vi "Actor Core.vi"(8 "error in":errorcluster, 11 "Nested in":refnum<class "FlatFieldUI.lvclass">) -> (0 "error out":errorcluster, 3 "Actor out":refnum<class "Actor.lvclass">)   [LabVIEW 2020, in "FlatFieldUI.lvlib" / "FlatFieldUI.lvclass"]
doc: "(<B>Filename</B>: Actor Framework.lvlib:Actor.lvclass:Actor Core.vi)\n\nReceives messages to the actor, reacts to them, and initiates any error handling that may shut the actor down.\n\nDescendant classes may override this VI to append parallel tasks for the actor to complete while it handles messages. Overrides use the Call Parent Method node."
uses:
  FlatFieldUI.lvclass
  <vilib>/ActorFramework/Actor/Actor.lvclass
  Displayer/Displayer/FlatField Method.ctl
  FlatFieldUI.lvclass/FlatFieldUI.ctl
  Hardware Abstraction Layer/Component/Device/Device/DataExchange.ctl
  Interface/DataListener Messages/OnDataChange Msg/OnDataChange Msg.lvclass/OnDataChange Msg.ctl
  <vilib>/ActorFramework/Message Enqueuer/Message Enqueuer.lvclass/Message Enqueuer.ctl
  <vilib>/ActorFramework/Message Enqueuer/Enqueue.vi
  Interface/DataListener Messages/OnDataChange Msg/OnDataChange Msg.lvclass
  C:/Program Files/National Instruments/LabVIEW 2020/vi.lib/ActorFramework/Message/Message.lvclass
  <vilib>/ActorFramework/Stop Msg/Stop Msg.lvclass
  <vilib>/ActorFramework/Message Priority Queue/Priority Enqueue.vi
  Hardware Abstraction Layer/Component/GenericActor/GenericActor/GenericController.lvclass
  Interface/DataListener/DataListener.lvclass
  <vilib>/vision/NI_Vision_Development_Module.lvlib
  E:/Development/DevHardSoftware/MicroscopyFramework/Model/Hardware Abstraction Layer/Component/GenericActor/GenericActor/GenericController.lvclass
  C:/Program Files/National Instruments/LabVIEW 2020/vi.lib/ActorFramework/Actor/Actor.lvclass
  E:/Development/DevHardSoftware/MicroscopyFramework/Interface/DataGenerator/DataGenerator.lvclass
  E:/Development/DevHardSoftware/MicroscopyFramework/Interface/DataListener/DataListener.lvclass
  E:/Development/DevHardSoftware/MicroscopyFramework/Interface/ErrorHandler/ErrorHandler.lvclass
  E:/Development/DevHardSoftware/MicroscopyFramework/Model/Logic Layer/FlatFieldUI/FlatFieldUI.lvclass
panel:
  in  "ZoomToFit":bool
  in  "Plot":bool
  in  "FlatFieldPath":path
  in  "DarkFieldPath":path
  in  "Save FlatField Image":bool
  in  "Save DarkField Image":bool
  in  "Method":T1 items=["Average", "Median"]
  out "XY Graph":cluster{"X":dbl, "Y":dbl}[](graph)
  in  "Show FlatField Image":bool
  in  "Show DarkField Image":bool
  out "Frames/Dark Field":dbl
  out "Frames/Flat-Field":dbl
  in  "Frames/Flat-Field":dbl
  in  "Frames/Dark Field":dbl
  in  "TakeFlatFieldImage":bool
  in  "TakeDarkFieldImage":bool
  out "RawImage":T2(plugin-control)
  in  "Flat-Field":bool
  # "* Please Take DarkField & Flat Field Images In Live Mode\n* You need to save the DarkField/FlatField images manually for post-processing"
  # "/"
  # "1."
  # "/"
  # "2."
  # "3."
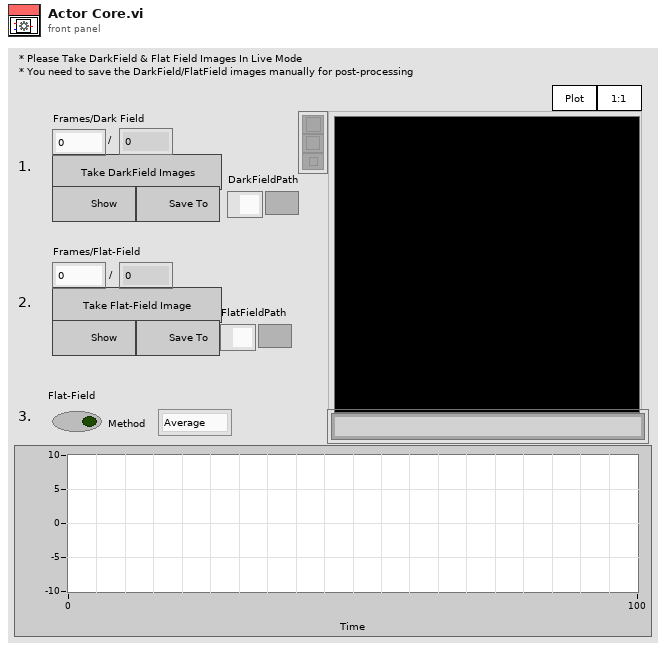
[diagram p1: front panel]
types:
  T1 = typedef "FlatFieldUI.lvlib/FlatFieldUI.lvclass/FlatField Method.ctl" = i32
  T2 = typedef "IMAQ Image.ctl" = refnum<image>
  T3 = cluster{"Stop":refnum<user-event>, "Image":refnum<user-event>}
  T4 = typedef "DataListener.lvclass/DataExchange.ctl" = cluster{"Source":string, "Destination":string, "Description":string, "value":variant}
  T5 = cluster{"Global Rectangle":i32[], "Contours":cluster{"Contour Type":u32, "ROI Type":u32, "Points":i32[]}[]}
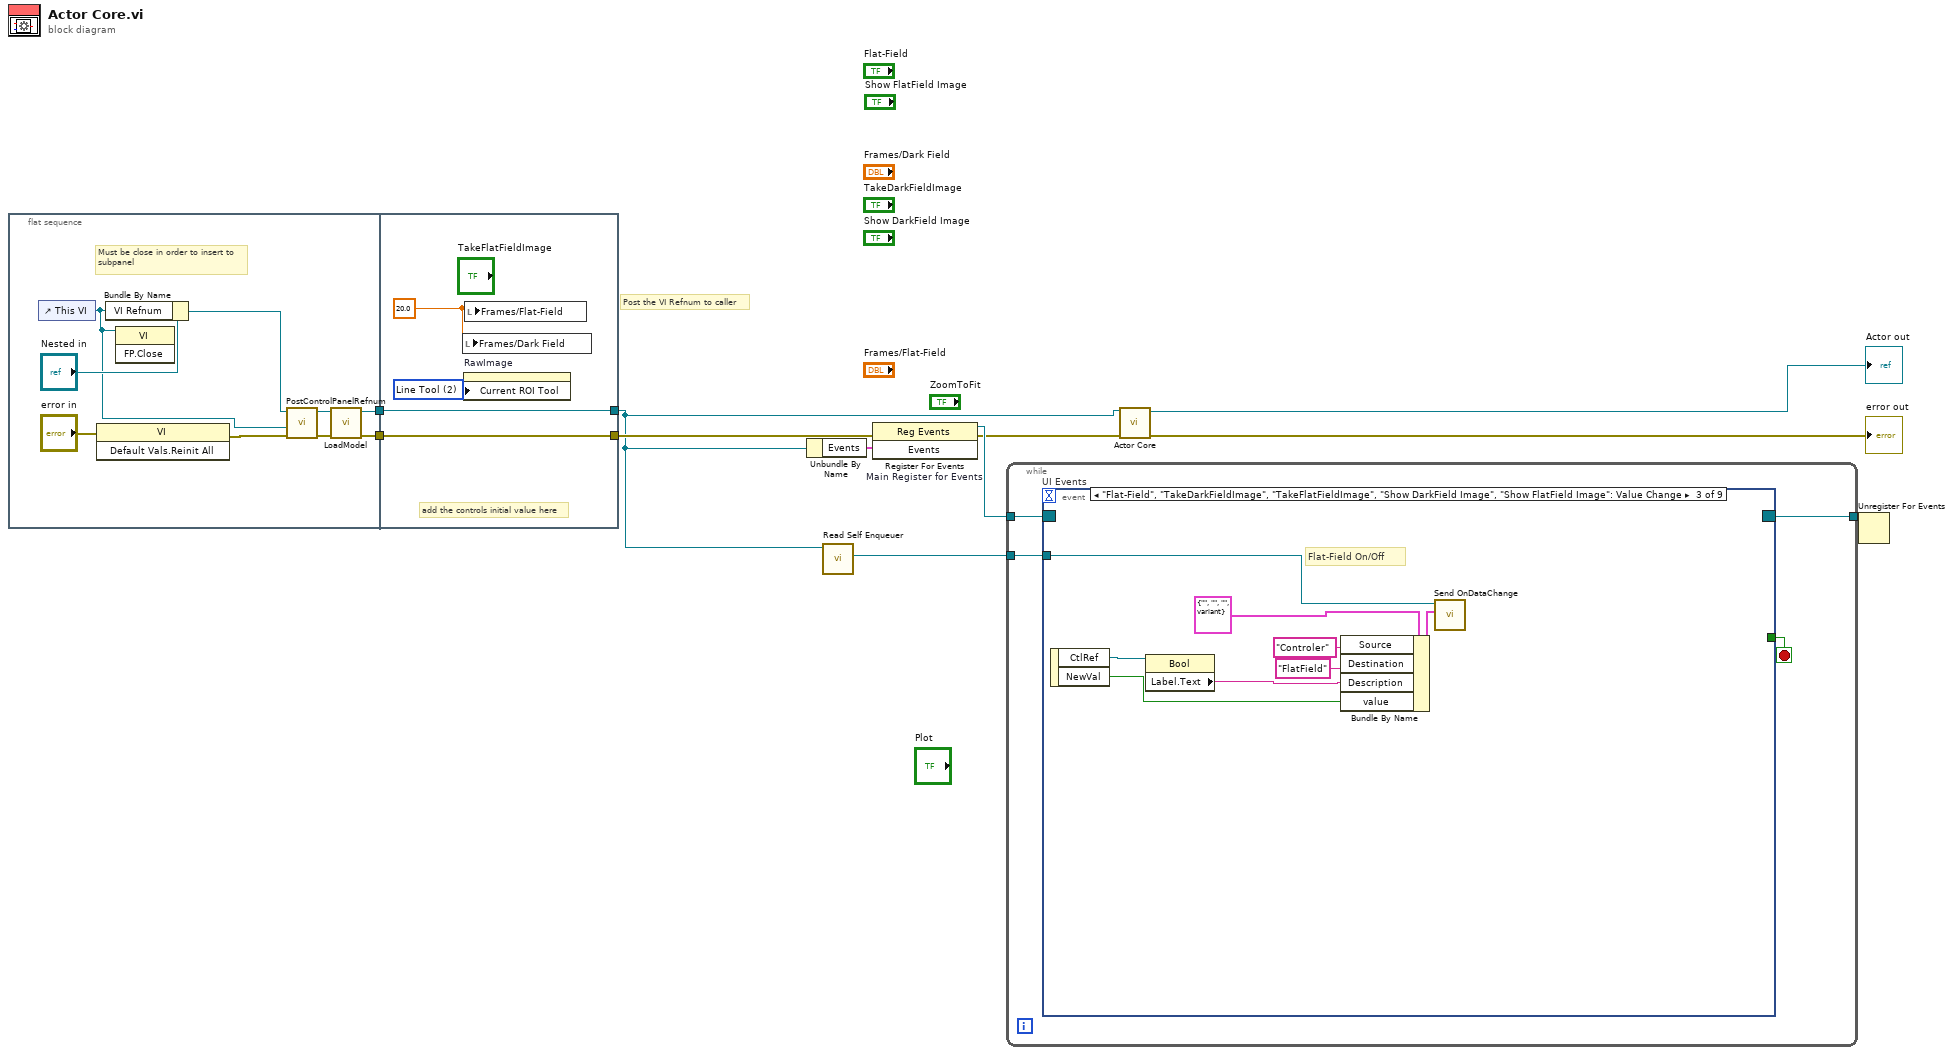
[diagram p0: block diagram]
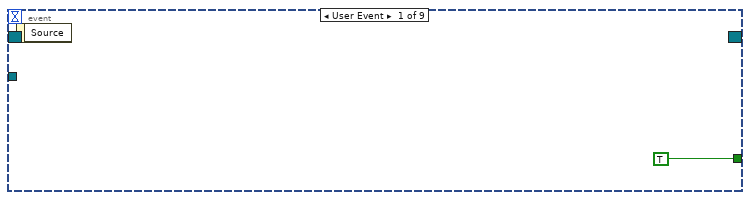
[diagram p2: hidden frame]
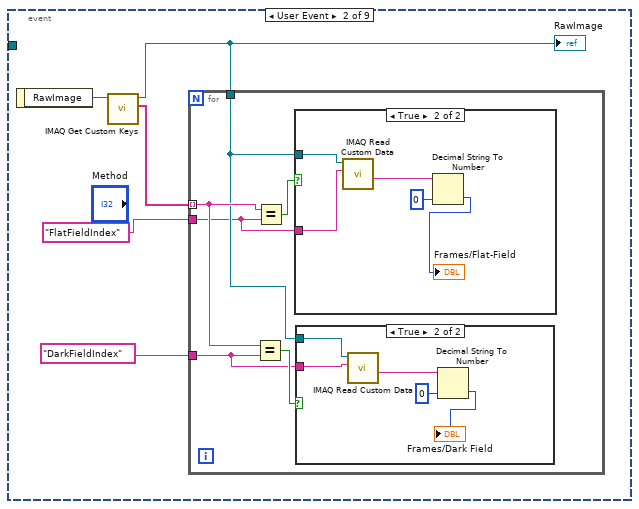
[diagram p3: hidden frame]
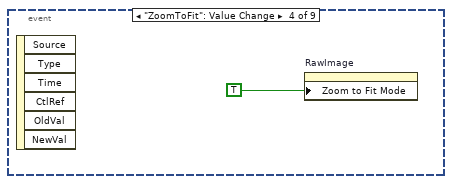
[diagram p6: hidden frame]
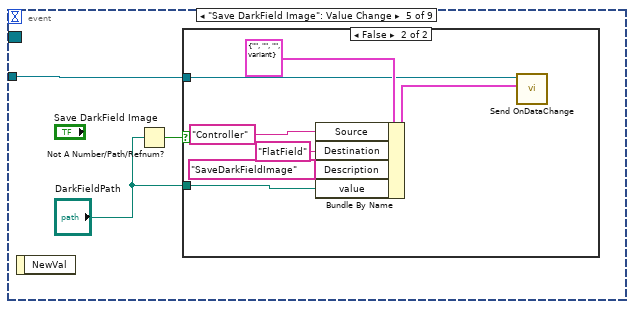
[diagram p7: hidden frame]
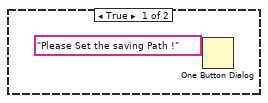
[diagram p8: hidden frame]
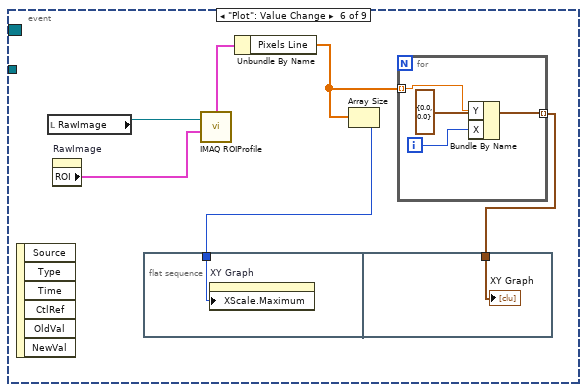
[diagram p9: hidden frame]
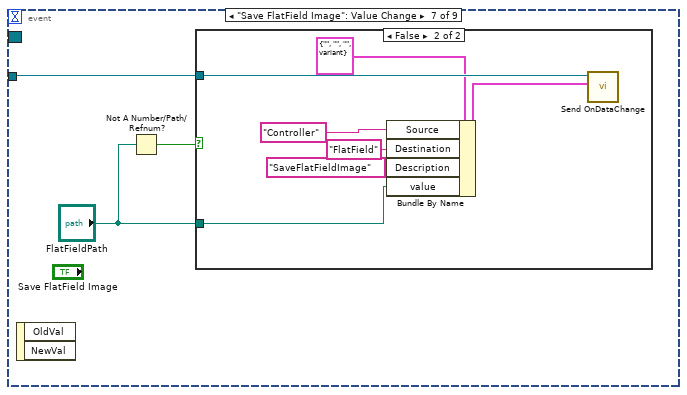
[diagram p10: hidden frame]
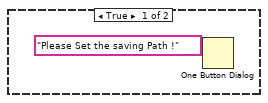
[diagram p11: hidden frame]
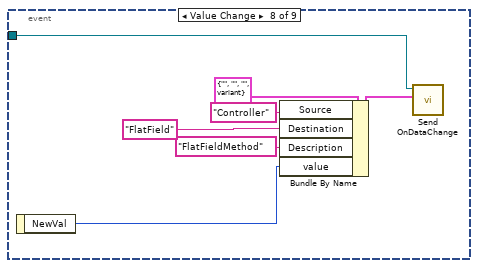
[diagram p12: hidden frame]
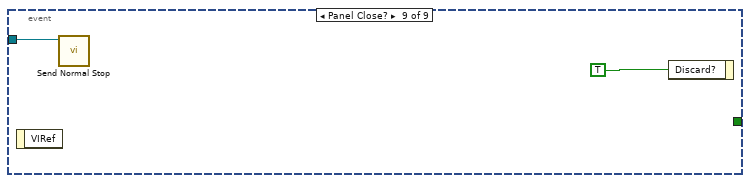
[diagram p13: hidden frame]
diagram:
  # "Post the VI Refnum to caller"
  n1 = flat-sequence {
    tunnel: [w14] -> w5
    tunnel: [w12] -> w4
    tunnel: [w23] -> w2
    tunnel: [w24] -> w3
    tunnel: w5 -> [w24]
    tunnel: w4 -> [w23]
    frame #0 {
      # "Must be close in order to insert to\nsubpanel"
      n2 = control-ref of="This VI"() -> (w15:refnum<vi>)
      n3 = invoke class="VI" method="Default Vals.Reinit All"(error in="error in") -> (error out=w18:errorcluster)  [unwired: 2 in, 2 out]
      n4 = Bundle By Name(cluster="Nested in", "VI Refnum"=w15) -> (w16:refnum<class "FlatFieldUI.lvclass">)
      n5 = invoke class="VI" method="FP.Close"(reference=w15) -> ()  [unwired: 2 in, 3 out]
      n6 = call-dynamic "PostControlPanelRefnum.vi"("error in (no error)"=w18, "VI Refnum"=w15, "GRMActor in"=w16) -> ("error out"=w17:errorcluster, "GRMActor out"=w13:refnum<class "FlatFieldUI.lvclass">)  [unwired: 7 in]
      n7 = call-dynamic "LoadModel.vi"("error in (no error)"=w17, "GRMActor in"=w13) -> ("error out"=w14:errorcluster, "GRMActor out"=w12:refnum<class "FlatFieldUI.lvclass">)  [unwired: 8 in]
    }
    frame #1 {
      w21 = u32 2 items=["Zoom Tool"=8, "Selection Tool"=0, "Pan Tool"=9, "Point Tool"=1, "Line Tool"=2, "Rectangle Tool"=3, "Rotated Rectangle Tool"=12, "Polyline Tool"=10, "Polygon Tool"=5, "Freehand Tool"=11, "Closed Freehand Tool"=6, "Ellipse Tool"=4, "Annulus Tool"=7] ("Current ROI Tool")
      w22 = 20.0 ("Frames/Flat-Field")
      # "add the controls initial value here"
      n8 = local write "Frames/Dark Field"(w22) -> ()
      n9 = property on="RawImage" class="ImageControl"("Current ROI Tool"=w21) -> ()  [unwired: 2 in, 2 out]
      n10 = local write "Frames/Flat-Field"(w22) -> ()
    }
  }
  n11 = Unbundle By Name(w2) -> ("Events"=w8:T3)
  n12 = call <vilib>:"Read Self Enqueuer.vi"("Actor"=w2) -> ("Self Enqueuer"=w1:refnum<class "Message Enqueuer.lvclass">)  [unwired: 10 in]
  n13 = register-events "Main Register for Events"(error in=w3, w8) -> (reference out=w9:refnum<event-registration>, error out=w6:errorcluster)  [unwired: 1 in]
  n14 = while {
    tunnel: w9 -> [w28]
    tunnel: [w26] -> w7
    tunnel: w1 -> [w25]
    stop <- w27 stop-if-true
    n15 = event "UI Events" shown="[2] \"Flat-Field\", \"TakeDarkFieldImage\", \"TakeFlatFieldImage\", \"Show DarkField Image\", \"Show FlatField Image\": Value Change" {
      selector: w28 -> [_ _ _ _ _ _ _ _ _]
      dyn-events: [_ _ _ _ _ _ _ _ _] -> w26
      timeout: _ -> [_ _ _ _ _ _ _ _ _]
      tunnel: [TRUE _ _ _ _ _ _ _ _] -> w27
      tunnel: w25 -> [_ _ w58 _ w62 _ w85 w100 w101]
      event User Event {
        n16 = event-data() -> ()  [unwired: 1 in, 1 out]
      }
      event User Event {
        n17 = event-data() -> ("RawImage"=w34:T2)  [unwired: 1 in]
        n18 = call "IMAQ Get Custom Keys"("Image"=w34) -> ("Keys"=w33:string[], "Image (duplicate)"=w30:T2)  [unwired: 7 in, 2 out]
        "RawImage" <- w30
        n19 = for {
          tunnel: w33 -> [w40] mode=indexing
          tunnel: "FlatFieldIndex" ("Key") -> [w36]
          tunnel: "DarkFieldIndex" ("Key") -> [w35]
          tunnel: w30 -> [w37]
          n20 = Equal?(x=w40, y=w35) -> (x = y?=w38:bool)
          n21 = Equal?(x=w40, y=w36) -> (x = y?=w39:bool)
          n22 = case shown="True" w39 {
            tunnel: w37 -> [_ w48]
            tunnel: w36 -> [_ w47]
            frame False {
            }
            frame True {
              n23 = call "IMAQ Read Custom Data"("Key"=w47, "Image"=w48) -> ("Custom Data Out"=w50:string)  [unwired: 7 in, 2 out]
              n24 = Decimal String To Number(string=w50, default (0L)=0 ("default (0 I32)")) -> (number=→"Frames/Flat-Field":i32)  [unwired: 1 in, 1 out]
            }
          }
          n25 = case shown="True" w38 {
            tunnel: w37 -> [_ w43]
            tunnel: w35 -> [_ w42]
            frame False {
            }
            frame True {
              n26 = call "IMAQ Read Custom Data"("Key"=w42, "Image"=w43) -> ("Custom Data Out"=w44:string)  [unwired: 7 in, 2 out]
              n27 = Decimal String To Number(string=w44, default (0L)=0 ("default (0 I32)")) -> (number=→"Frames/Dark Field":i32)  [unwired: 1 in, 1 out]
            }
          }
        }
      }
      event "Flat-Field", "TakeDarkFieldImage", "TakeFlatFieldImage", "Show DarkField Image", "Show FlatField Image": Value Change {
        # "Flat-Field On/Off"
        n28 = event-data() -> ("CtlRef"=w57:refnum<vi>, "NewVal"=w51:bool)  [unwired: 1 in]
        n29 = property class="Bool"(reference=w57) -> ("Label.Text"=w52:string)  [unwired: 1 in, 2 out]
        n30 = Bundle By Name(cluster=T4 {"Source"="", "Destination"="", "Description"="", "value"=variant} ("DataExchange"), "Source"="Controler", "Destination"="FlatField", "Description"=w52, "value"=w51) -> (w55:T4)
        n31 = call "Send OnDataChange.vi"("DataExchange"=w55, "Message Enqueuer"=w58) -> ()  [unwired: 8 in, 2 out]
      }
      event "ZoomToFit": Value Change {
        n32 = event-data() -> ()  [unwired: 1 in, 6 out]
        n33 = property on="RawImage" class="ImageControl"("Zoom to Fit Mode"=TRUE) -> ()  [unwired: 2 in, 2 out]
      }
      event "Save DarkField Image": Value Change {
        n34 = event-data() -> ()  [unwired: 1 in, 1 out]
        n35 = Not A Number/Path/Refnum?(number/path/refnum="DarkFieldPath") -> (NaN/Path/Refnum?=w61:bool)
        n36 = case shown="False" w61 {
          tunnel: w62 -> [_ w65]
          tunnel: "DarkFieldPath" -> [_ w64]
          frame True {
            n37 = One Button Dialog(message="Please Set the saving Path !") -> ()  [unwired: 1 in, 1 out]
          }
          frame False {
            n38 = Bundle By Name(cluster=T4 {"Source"="", "Destination"="", "Description"="", "value"=variant} ("DataExchange"), "Source"="Controller", "Destination"="FlatField", "Description"="SaveDarkFieldImage", "value"=w64) -> (w69:T4)
            n39 = call "Send OnDataChange.vi"("DataExchange"=w69, "Message Enqueuer"=w65) -> ()  [unwired: 8 in, 2 out]
          }
        }
      }
      event "Plot": Value Change {
        n40 = event-data() -> ()  [unwired: 1 in, 6 out]
        n41 = local read "RawImage"() -> (w76:T2)
        n42 = property on="RawImage" class="ImageControl"() -> ("ROI"=w75:T5)  [unwired: 2 in, 2 out]
        n43 = flat-sequence {
          tunnel: w73 -> [w81]
          tunnel: w71 -> [w82]
          frame #0 {
            n44 = property on="XY Graph" class="XYGraph (strict)"("XScale.Maximum"=w81) -> ()  [unwired: 2 in, 2 out]
          }
          frame #1 {
            "XY Graph" <- w82
          }
        }
        n45 = call "IMAQ ROIProfile"("ROI Descriptor"=w75, "Image"=w76) -> ("ROI Graph"=w74:cluster{"x0":sgl, "dx":sgl, "Pixels Line":sgl[]})  [unwired: 2 in, 4 out]
        n46 = Unbundle By Name(w74) -> ("Pixels Line"=w72:sgl[])
        n47 = Array Size(array=w72) -> (size(s)=w73:i32)
        n48 = for {
          tunnel: w72 -> [w77] mode=indexing
          tunnel: [w79] -> w71 mode=indexing
          i -> [w78]
          n49 = Bundle By Name(cluster=cluster{"X":dbl, "Y":dbl} {"X"=0.0, "Y"=0.0}, "Y"=w77, "X"=w78) -> (w79:cluster{"X":dbl, "Y":dbl})
        }
      }
      event "Save FlatField Image": Value Change {
        n50 = event-data() -> ()  [unwired: 1 in, 2 out]
        n51 = Not A Number/Path/Refnum?(number/path/refnum="FlatFieldPath") -> (NaN/Path/Refnum?=w83:bool)
        n52 = case shown="False" w83 {
          tunnel: w85 -> [_ w93]
          tunnel: "FlatFieldPath" -> [_ w87]
          frame True {
            n53 = One Button Dialog(message="Please Set the saving Path !") -> ()  [unwired: 1 in, 1 out]
          }
          frame False {
            n54 = Bundle By Name(cluster=T4 {"Source"="", "Destination"="", "Description"="", "value"=variant} ("DataExchange"), "Source"="Controller", "Destination"="FlatField", "Description"="SaveFlatFieldImage", "value"=w87) -> (w91:T4)
            n55 = call "Send OnDataChange.vi"("DataExchange"=w91, "Message Enqueuer"=w93) -> ()  [unwired: 8 in, 2 out]
          }
        }
      }
      event Value Change {
        n56 = event-data() -> ("NewVal"=w97:T1)  [unwired: 1 in]
        n57 = Bundle By Name(cluster=T4 {"Source"="", "Destination"="", "Description"="", "value"=variant} ("DataExchange"), "Source"="Controller", "Destination"="FlatField", "Description"="FlatFieldMethod", "value"=w97) -> (w98:T4)
        n58 = call "Send OnDataChange.vi"("DataExchange"=w98, "Message Enqueuer"=w100) -> ()  [unwired: 8 in, 2 out]
      }
      event Panel Close? {
        n59 = event-data() -> ()  [unwired: 1 in, 1 out]
        n60 = call <vilib>:"Send Normal Stop.vi"("Message Enqueuer"=w101) -> ()  [unwired: 10 in, 1 out]
        n61 = event-data("Discard?"=TRUE) -> ()  [unwired: 1 in, 1 out]
      }
    }
  }
  n62 = call-parent "Actor Core.vi"("error in"=w6, "GenericController in"=w2) -> ("error out"=→"error out":errorcluster, "Actor out"=→"Actor out":refnum<class "Actor.lvclass">)  [unwired: 8 in]
  n63 = Unregister For Events(event registration refnum=w7) -> ()  [unwired: 1 in, 1 out]
